vi "ni_home.vi"(8 "error in":errorcluster) -> (0 "error out":errorcluster)   [LabVIEW 2011]
uses:
  <vilib>/Motion/FlexMotion/CustomControls/CustomControls.llb/Axis # (8 axes).flx
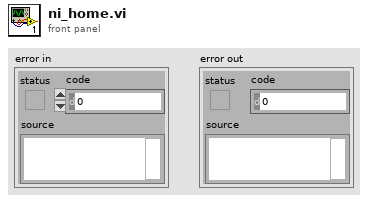
[diagram p1: front panel]
types:
  T1 = typedef "Board Id" = u8
  T2 = enum16{"Home", "Index", "Center", "Forward Limit", "Reverse Limit", "Run Sequence"}
  T3 = typedef "Axis # (8 axes).flx" = cluster{"1":bool, "2":bool, "3":bool, "4":bool, "5":bool, "6":bool, "7":bool, "8":bool}
  T4 = typedef "AxisOrVectorSpaceControl To Control.flx" = u16
  T5 = typedef "Bd Id Out" = u8
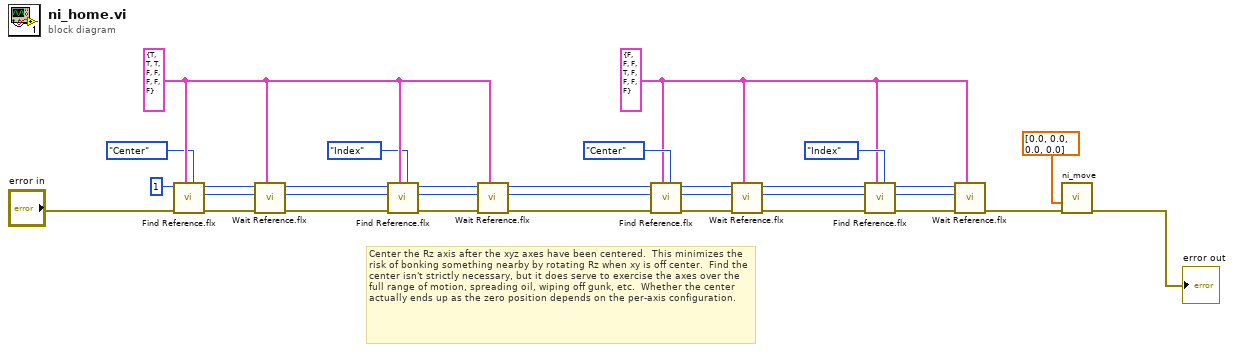
[diagram p0: block diagram]
diagram:
  w17 = T3 {"1"=FALSE, "2"=FALSE, "3"=FALSE, "4"=TRUE, "5"=FALSE, "6"=FALSE, "7"=FALSE, "8"=FALSE} ("Axis/VS Map (Disabled)")
  w16 = T3 {"1"=TRUE, "2"=TRUE, "3"=TRUE, "4"=FALSE, "5"=FALSE, "6"=FALSE, "7"=FALSE, "8"=FALSE} ("Axis/VS Map (Disabled)")
  # "Center the Rz axis after the xyz axes have been centered.  This minimizes the risk of bonking something nearby by rotating Rz when xy is off center.  Find the center isn't strictly necessary, but it does serve to exercise the axes over the full range of motion, spreading oil, wiping off gunk, etc.  Whether the center actually ends up as the zero position depends on the per-axis configuration."
  n1 = call <vilib>:"Find Reference.flx"("Search Type"=T2."Center", "Axis/VS Map (Disabled)"=w16, "error in (no error)"="error in", "Board ID"=T1 1) -> ("error out"=w4:errorcluster, "Axis or Vector Space Output"=w7:T4, "Bd ID Out"=w6:T5)  [unwired: 5 in]
  n2 = call <vilib>:"Wait Reference.flx"("Axis/VS Map (Disabled)"=w16, "error in (no error)"=w4, "Axis or Vector Space"=w7, "Board ID"=w6) -> ("error out"=w10:errorcluster, "Axis or Vector Space Output"=w15:T4, "Bd ID Out"=w14:T5)  [unwired: 4 in, 1 out]
  n3 = call <vilib>:"Find Reference.flx"("Search Type"=T2."Index", "Axis/VS Map (Disabled)"=w16, "error in (no error)"=w10, "Axis or Vector Space"=w15, "Board ID"=w14) -> ("error out"=w11:errorcluster, "Axis or Vector Space Output"=w13:T4, "Bd ID Out"=w12:T5)  [unwired: 4 in]
  n4 = call <vilib>:"Wait Reference.flx"("Axis/VS Map (Disabled)"=w16, "error in (no error)"=w11, "Axis or Vector Space"=w13, "Board ID"=w12) -> ("error out"=w31:errorcluster, "Axis or Vector Space Output"=w30:T4, "Bd ID Out"=w29:T5)  [unwired: 4 in, 1 out]
  n5 = call <vilib>:"Find Reference.flx"("Search Type"=T2."Center", "Axis/VS Map (Disabled)"=w17, "error in (no error)"=w31, "Axis or Vector Space"=w30, "Board ID"=w29) -> ("error out"=w28:errorcluster, "Axis or Vector Space Output"=w26:T4, "Bd ID Out"=w27:T5)  [unwired: 4 in]
  n6 = call <vilib>:"Wait Reference.flx"("Axis/VS Map (Disabled)"=w17, "error in (no error)"=w28, "Axis or Vector Space"=w26, "Board ID"=w27) -> ("error out"=w23:errorcluster, "Axis or Vector Space Output"=w18:T4, "Bd ID Out"=w19:T5)  [unwired: 4 in, 1 out]
  n7 = call <vilib>:"Find Reference.flx"("Search Type"=T2."Index", "Axis/VS Map (Disabled)"=w17, "error in (no error)"=w23, "Axis or Vector Space"=w18, "Board ID"=w19) -> ("error out"=w22:errorcluster, "Axis or Vector Space Output"=w20:T4, "Bd ID Out"=w21:T5)  [unwired: 4 in]
  n8 = call <vilib>:"Wait Reference.flx"("Axis/VS Map (Disabled)"=w17, "error in (no error)"=w22, "Axis or Vector Space"=w20, "Board ID"=w21) -> ("error out"=w3:errorcluster)  [unwired: 4 in, 3 out]
  n9 = call "ni_move.vi"("error in"=w3, "Axis positions"=dbl[] [0.0, 0.0, 0.0, 0.0]) -> ("error out"=→"error out":errorcluster)  [unwired: 9 in]
